vi "HealthAndStatusTest.vi"() -> ()   [LabVIEW 2016]
uses:
  <vilib>/FPGAPlugInAG/cRIO-9038/niLvFpga_Open_cRIO-9038.vi
  <vilib>/rvi/interface/common/dynamic/niFpgaDynamicAddResources.vi
  <vilib>/FPGAPlugInAG/Dynamic/niLvFpga_Abort_Dynamic.vi
  <vilib>/FPGAPlugInAG/Dynamic/niLvFpga_Run_Dynamic.vi
  <vilib>/Utility/error.llb/Error Cluster From Error Code.vi
  <vilib>/rvi/errors/niLvFpgaAdjustHostInterfaceError.vi
  <vilib>/FPGAPlugInAG/Dynamic/niLvFpga_Close_Dynamic.vi
  <vilib>/rvi/interface/nirviOpenFPGA/nirviOpenFPGA.xnode
  FPGA Bitfiles/healthAndStatusTest.lvbitx
  FPGA/healthAndStatusTest.vi
  <vilib>/rvi/interface/nirviMethod/nirviMethod.xnode
  <vilib>/rvi/interface/nirviReadWriteControl/nirviReadWriteControl.xnode
  <vilib>/rvi/interface/nirviCloseFPGA/nirviCloseFPGA.xnode
  NiFpgaLv.dll
  <vilib>/rvi/interface/Simulation/niFpgaSimulationCallBeginRW.vi
  <vilib>/FPGAPlugInAG/Dynamic/niLvFpga_WriteFifo_Dynamic.vi
  <vilib>/rvi/errors/niLvFpgaMergeErrorWithErrorCode.vi
  <vilib>/FPGAPlugInAG/Dynamic/niLvFpga_ReadFifo_Dynamic.vi
panel:
  in  "Stop":bool
  out "Value":u32
  in  "Bit":i16
  in  "Set Bit":bool
  in  "Clear":bool
  in  "Sub 1":bool
  in  "Add 1":bool
  in  "Set":bool
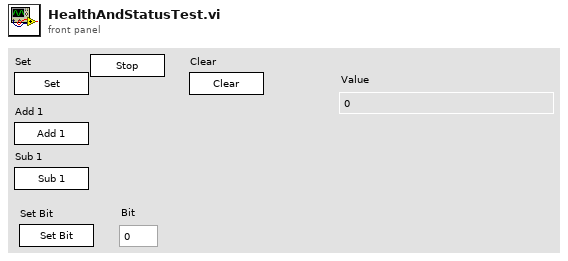
[diagram p1: front panel]
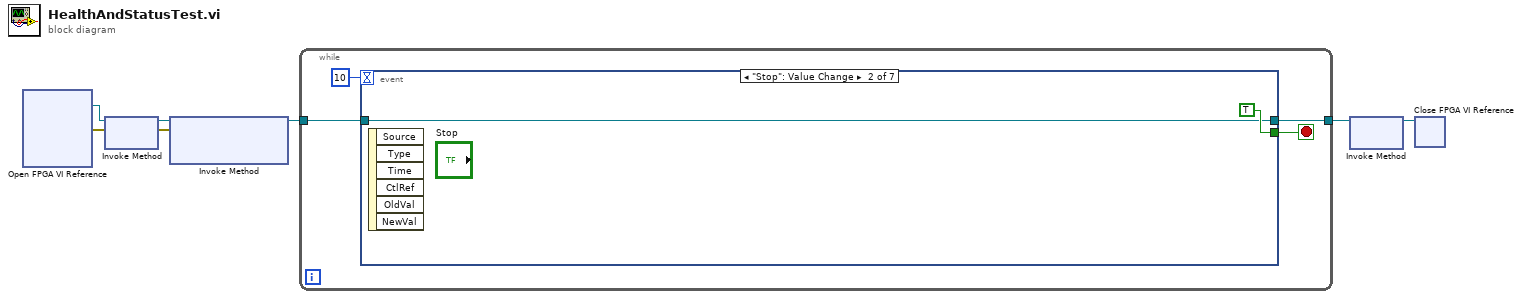
[diagram p0: block diagram]
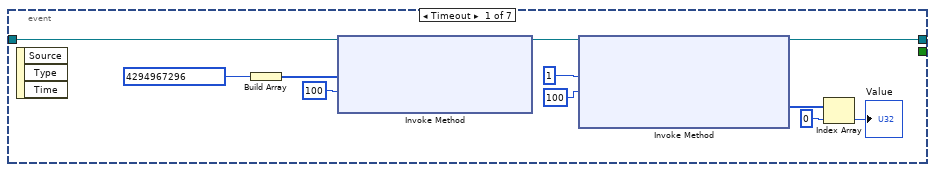
[diagram p2: hidden frame]
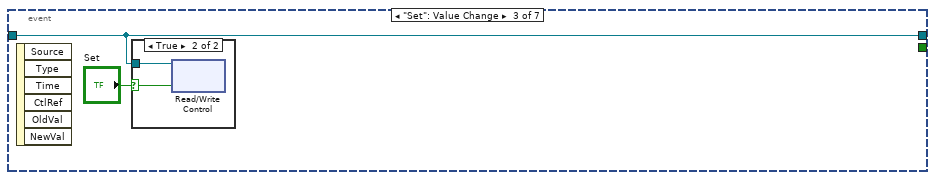
[diagram p3: hidden frame]
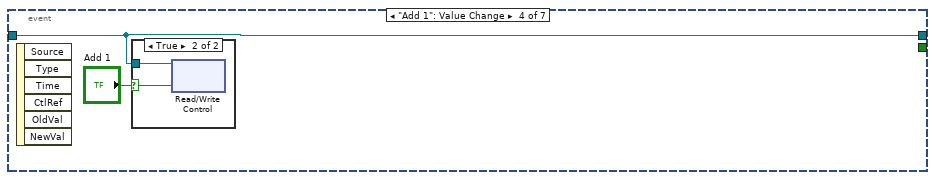
[diagram p5: hidden frame]
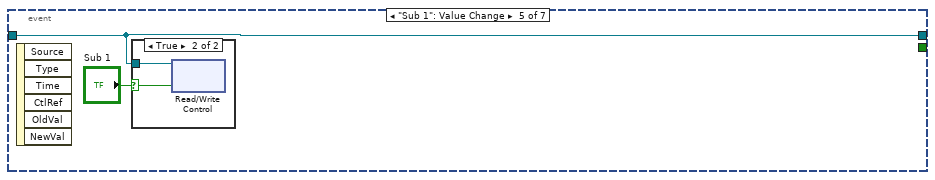
[diagram p7: hidden frame]
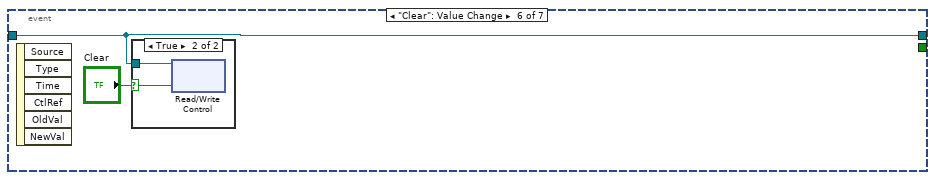
[diagram p9: hidden frame]
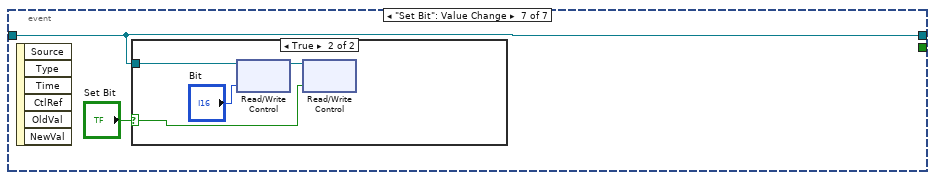
[diagram p11: hidden frame]
diagram:
  n1 = xnode "Open FPGA VI Reference"() -> ("FPGA VI Reference Out"=w7:refnum<k20>, "error out"=w5:errorcluster)  [unwired: 2 in]
  n2 = xnode "Invoke Method"("FPGA VI Reference In"=w7, "error in"=w5) -> ("FPGA VI Reference Out"=w6:refnum<k20>, "error out"=w4:errorcluster)
  n3 = xnode "Invoke Method"("FPGA VI Reference In"=w6, "error in"=w4) -> ("FPGA VI Reference Out"=w2:refnum<k20>)  [unwired: 1 in, 1 out]
  n4 = while {
    tunnel: w2 -> [w10]
    tunnel: [w8] -> w1
    stop <- w11 stop-if-true
    n5 = event shown="[1] \"Stop\": Value Change" {
      selector: _ -> [_ _ _ _ _ _ _]
      dyn-events: _ -> [_ _ _ _ _ _ _]
      timeout: 10 -> [_ _ _ _ _ _ _]
      tunnel: [_ TRUE _ _ _ _ _] -> w11
      tunnel: w10 -> [w22 w23 w25 w29 w33 w37 w41]
      tunnel: [w12 w23 w25 w29 w33 w37 w41] -> w8
      event Timeout {
        n6 = event-data() -> ()  [unwired: 1 in, 3 out]
        n7 = Build Array(u64 4294967296) -> (w20:u64[])
        n8 = xnode "Invoke Method"("FPGA VI Reference In"=w22, "Data"=w20, "Timeout (ms)"=100) -> ("FPGA VI Reference Out"=w19:refnum<k20>)  [unwired: 1 in, 2 out]
        n9 = xnode "Invoke Method"("FPGA VI Reference In"=w19, "Number of Elements"=u32 1, "Timeout (ms)"=100) -> ("FPGA VI Reference Out"=w12:refnum<k20>, "Data"=w15:u32[])  [unwired: 1 in, 2 out]
        n10 = Index Array(array=w15, index=0) -> (element=→"Value":u32)
      }
      event "Stop": Value Change {
        n11 = event-data() -> ()  [unwired: 1 in, 6 out]
      }
      event "Set": Value Change {
        n12 = event-data() -> ()  [unwired: 1 in, 6 out]
        n13 = case shown="True" "Set" {
          selector: "Set" -> [_ w27]
          tunnel: w25 -> [_ w28]
          frame False {
          }
          frame True {
            n14 = xnode "Read/Write Control"("FPGA VI Reference In"=w28, "Set0"=w27) -> ()  [unwired: 1 in, 2 out]
          }
        }
      }
      event "Add 1": Value Change {
        n15 = event-data() -> ()  [unwired: 1 in, 6 out]
        n16 = case shown="True" "Add 1" {
          selector: "Add 1" -> [_ w31]
          tunnel: w29 -> [_ w32]
          frame False {
          }
          frame True {
            n17 = xnode "Read/Write Control"("FPGA VI Reference In"=w32, "Add0"=w31) -> ()  [unwired: 1 in, 2 out]
          }
        }
      }
      event "Sub 1": Value Change {
        n18 = event-data() -> ()  [unwired: 1 in, 6 out]
        n19 = case shown="True" "Sub 1" {
          selector: "Sub 1" -> [_ w35]
          tunnel: w33 -> [_ w36]
          frame False {
          }
          frame True {
            n20 = xnode "Read/Write Control"("FPGA VI Reference In"=w36, "Sub0"=w35) -> ()  [unwired: 1 in, 2 out]
          }
        }
      }
      event "Clear": Value Change {
        n21 = event-data() -> ()  [unwired: 1 in, 6 out]
        n22 = case shown="True" "Clear" {
          selector: "Clear" -> [_ w39]
          tunnel: w37 -> [_ w40]
          frame False {
          }
          frame True {
            n23 = xnode "Read/Write Control"("FPGA VI Reference In"=w40, "Clear"=w39) -> ()  [unwired: 1 in, 2 out]
          }
        }
      }
      event "Set Bit": Value Change {
        n24 = event-data() -> ()  [unwired: 1 in, 6 out]
        n25 = case shown="True" "Set Bit" {
          selector: "Set Bit" -> [_ w43]
          tunnel: w41 -> [_ w46]
          frame False {
          }
          frame True {
            n26 = xnode "Read/Write Control"("FPGA VI Reference In"=w46, "Bit"="Bit") -> ("FPGA VI Reference Out"=w45:refnum<k20>)  [unwired: 1 in, 1 out]
            n27 = xnode "Read/Write Control"("FPGA VI Reference In"=w45, "SetBit"=w43) -> ()  [unwired: 1 in, 2 out]
          }
        }
      }
    }
  }
  n28 = xnode "Invoke Method"("FPGA VI Reference In"=w1) -> ("FPGA VI Reference Out"=w3:refnum<k20>)  [unwired: 1 in, 1 out]
  n29 = xnode "Close FPGA VI Reference"("FPGA VI Reference In"=w3) -> ()  [unwired: 1 in, 1 out]
